vi "Write to Coils DB.vi"(8 "error in (no error)":errorcluster, 9 "Values":bool[](array[boolean]), 10 "Modbus Address":u16, 11 "MB Cache in":refnum<class "MB Data Block.lvclass">) -> (0 "error out":errorcluster, 3 "MB Cache out":refnum<class "MB Data Block.lvclass">)   [LabVIEW 2018, in "MB PLC Client.lvlib" / "MB Data Block.lvclass"]
uses:
  MB Data Block.lvclass
  MB Data Block.lvclass/MB Data Block.ctl
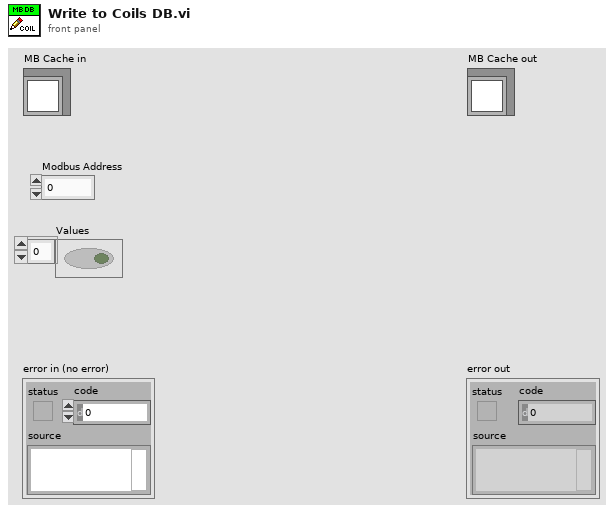
[diagram p1: front panel]
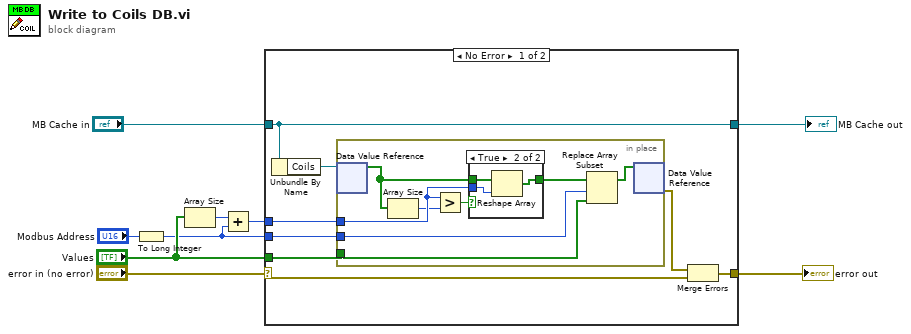
[diagram p0: block diagram]
diagram:
  n1 = To Long Integer(number="Modbus Address") -> (32bit integer=w5:i32)
  n2 = Array Size(array="Values") -> (size(s)=w6:i32)
  n3 = Add(x=w6, y=w5) -> (x+y=w4:i32)
  n4 = case shown="No Error" "error in (no error)" {
    selector: "error in (no error)" -> [w11 w31]
    tunnel: w4 -> [w17 _]
    tunnel: "Values" -> [w16 _]
    tunnel: [w12 w31] -> w2
    tunnel: w5 -> [w15 _]
    tunnel: "MB Cache in" -> [w14 w30]
    tunnel: [w14 w30] -> w1
    frame No Error {
      n5 = Unbundle By Name(w14) -> ("Coils"=w13:refnum<data-value>)
      n6 = in-place {
        in-place-border: w17 -> [w25]
        in-place-border: w16 -> [w24]
        in-place-border: w15 -> [w23]
        n7 = in-place-dvr #1(w13) -> (w19:bool[])  [unwired: 1 out]
        n8 = Array Size(array=w19) -> (size(s)=w21:i32)
        n9 = Greater?(x=w25, y=w21) -> (0:w22:bool)
        n10 = case shown="True" w22 {
          tunnel: w19 -> [w26 w29]
          tunnel: [w26 w28] -> w20
          tunnel: w25 -> [_ w27]
          frame False {
          }
          frame True {
            n11 = Reshape Array(w29, w27) -> (w28:bool[])
          }
        }
        n12 = Replace Array Subset(array=w20, new element=w24, index=w23) -> (w18:bool[])
        n13 = in-place-dvr #1(w18) -> (w10:errorcluster)  [unwired: 1 out]
      }
      n14 = Merge Errors(w10, w11) -> (w12:errorcluster)
    }
    frame Error {
    }
  }
  "error out" <- w2
  "MB Cache out" <- w1
